vi "Configure Trend Rate.vi"(0 "VISA resource name":refnum<visa-resource-name>, 5 "Enable Trend Rate Switching (False)":bool, 7 "Second Interval (4: 1min)":u16(ring)=4 items=["5s", "10s", "15s", "30s", "1min", "2min", "5min", "10min", "15min", "20min", "30min", "1h", "2h", "4h", "10h"], 11 "error in (no error)":errorcluster) -> (4 "VISA resource name out":refnum<visa-resource-name>, 15 "error out":errorcluster)   [LabVIEW 2020, in "Yokogawa GX Series.lvlib"]
doc: "Sets the trend interval switching.\n\nCommand: STrdRate\n\nNote: This VI does nothing when the instrument is GM10."
uses:
  <instrlib>/Yokogawa GX Series/Yokogawa GX Series.lvlib
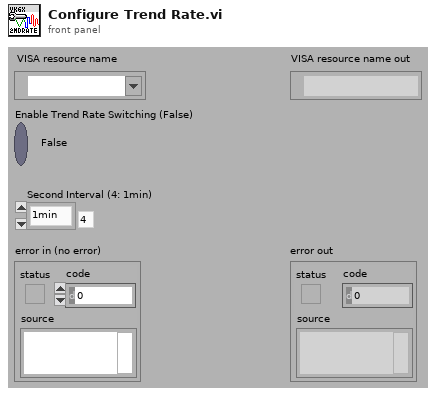
[diagram p1: front panel]
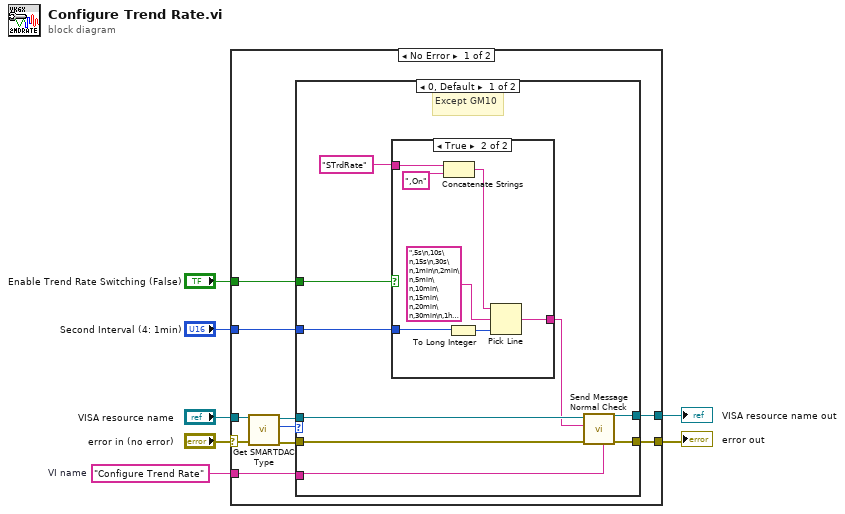
[diagram p0: block diagram]
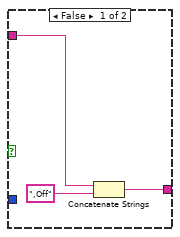
[diagram p2: hidden frame]
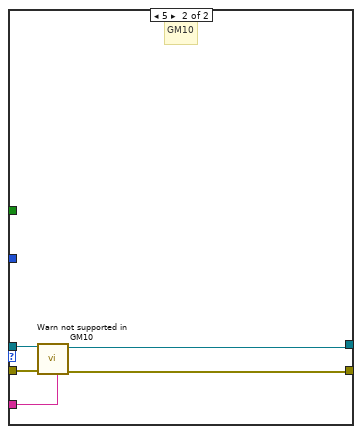
[diagram p3: hidden frame]
diagram:
  w6 = "Configure Trend Rate"  # VI name
  n1 = case shown="No Error" "error in (no error)" {
    selector: "error in (no error)" -> [w11 w42]
    tunnel: "VISA resource name" -> [w12 w43]
    tunnel: w6 -> [w17 _]
    tunnel: [w16 w43] -> w5
    tunnel: [w15 w42] -> w4
    tunnel: "Second Interval (4: 1min)" -> [w14 _]
    tunnel: "Enable Trend Rate Switching (False)" -> [w13 _]
    frame No Error {
      n2 = call <instrlib>:"Get SMARTDAC Type.vi"("error in (no error)"=w11, "VISA resource name"=w12) -> ("error out"=w9:errorcluster, "SMARTDAC+ Type"=w8:u16, "VISA resource name out"=w10:refnum<visa-resource-name>)  [unwired: 7 in]
      n3 = case shown="0, Default" w8 {
        tunnel: w10 -> [w26 w41]
        tunnel: w17 -> [w25 w37]
        tunnel: [w24 w39] -> w16
        tunnel: [w23 w38] -> w15
        tunnel: w14 -> [w22 _]
        tunnel: w13 -> [w20 _]
        tunnel: w9 -> [w19 w40]
        frame 0, Default {
          # "Except GM10"
          n4 = case shown="True" w20 {
            tunnel: "STrdRate" -> [w29 w34]
            tunnel: w22 -> [_ w30]
            tunnel: [w27 w36] -> w21
            frame False {
              n5 = Concatenate Strings(w29, ",Off") -> (w27:string)
            }
            frame True {
              n6 = Concatenate Strings(w34, ",On") -> (w32:string)
              n7 = To Long Integer(number=w30) -> (32bit integer=w31:i32)
              n8 = Pick Line(string ("")=w32, multi-line string=",5s\n,10s\n,15s\n,30s\n,1min\n,2min\n,5min\n,10min\n,15min\n,20min\n,30min\n,1h\n,2h\n,4h\n,10h", line index=w31) -> (output string=w36:string)
            }
          }
          n9 = call <instrlib>:"Send Message Normal Check.vi"("Source (\"\")"=w25, "error in (no error)"=w19, "Send Message (\"\")"=w21, "VISA resource name"=w26) -> ("error out"=w23:errorcluster, "VISA resource name out"=w24:refnum<visa-resource-name>)  [unwired: 2 in, 4 out]
        }
        frame 5 {
          # "GM10"
          n10 = call <instrlib>:"Warn not supported in GM10.vi"("Source (\"\")"=w37, "error in (no error)"=w40, "VISA resource name"=w41) -> ("error out"=w38:errorcluster, "VISA resource name out"=w39:refnum<visa-resource-name>)  [unwired: 7 in]
        }
      }
    }
    frame Error {
    }
  }
  "error out" <- w4
  "VISA resource name out" <- w5
